vi "Config Ackermann Frame.vi"(10 "subpanel to main command event":T1, 11 "main to subpanel command event reg":T2) -> ()   [LabVIEW 2017, in "NI_Robotics_Configure Steering Frame.lvlib" / "Ackermann Frame Subpanel.lvlib"]
uses:
  <vilib>/robotics/Dialog/Configure Steering Frame/Ackermann Frame Subpanel/Ackermann Frame Subpanel.lvlib
  <vilib>/robotics/Dialog/Configure Steering Frame/Main to Subpanel Command Event Reg.ctl
  <vilib>/robotics/Dialog/Configure Steering Frame/Main to Subpanel Command.ctl
  <vilib>/robotics/Steering/Steering Frame/NI_Robotics_Steering Frame.lvclass
  <vilib>/robotics/Dialog/Configure Steering Frame/Subpanel to Main Command Event.ctl
  <vilib>/robotics/Dialog/Configure Steering Frame/Subpanel to Main Command.ctl
  <vilib>/robotics/Dialog/Configure Steering Frame/Ackermann Frame Subpanel/FP Refs.ctl
  <vilib>/robotics/Steering/Ackermann Steering Frame/NI_Robotics_Ackermann Steering Frame.lvclass
  c:/Program Files (x86)/National Instruments/LabVIEW 2017/vi.lib/robotics/Steering/Steering Frame/NI_Robotics_Steering Frame.lvclass
  <vilib>/robotics/Steering/Steering Frame/NI_Robotics_Steering Frame.lvclass/NI_Robotics_Steering Frame.ctl
  <vilib>/robotics/Steering/Wheel/NI_Robotics_Wheel.lvclass/NI_Robotics_Wheel.ctl
  <vilib>/robotics/Steering/Ackermann Steering Frame/NI_Robotics_Ackermann Steering Frame.lvclass/NI_Robotics_Ackermann Steering Frame.ctl
  <vilib>/robotics/Dialog/Configure Steering Frame/Send Update Picture Command.vi
  <vilib>/robotics/Steering/Ackermann Steering Frame/Set Wheel Separations.vi
  <vilib>/robotics/Dialog/Configure Steering Frame/Generate Subpanel to Main Event.vi
  <vilib>/Utility/error.llb/Clear Errors.vi
  <vilib>/robotics/Steering/Ackermann Steering Frame/Wheel Separation to Frame Positions.vi
  <vilib>/robotics/Steering/Steering Frame/Reposition Wheels.vi
  <vilib>/robotics/Steering/Wheel/Update Steering to Wheel Frame Transform.vi
  <vilib>/Analysis/coordinate.llb/Wrap Angle.vi
  <vilib>/Analysis/coordinate.llb/Wrap Angle (scalar).vi
  <vilib>/robotics/Steering/Steering Frame/Set All Gear Ratio.vi
  <vilib>/robotics/Steering/Steering Frame/Set All Wheel Radius.vi
  <vilib>/robotics/Dialog/Configure Steering Frame/NI_Robotics_Configure Steering Frame.lvlib
panel:
  in  "Wheel Separation Length":dbl
  in  "Wheel Separation Width":dbl
  in  "Gear Ratio":dbl
  in  "Wheel Radius":dbl
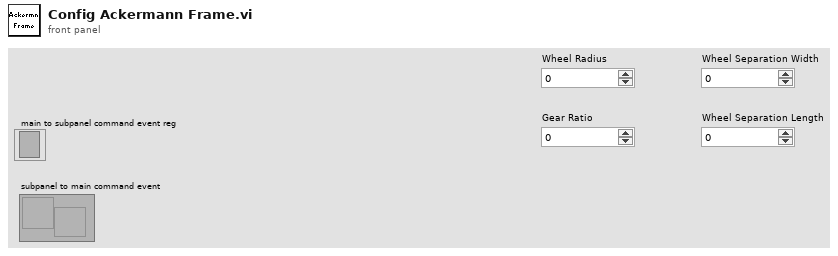
[diagram p1: front panel]
types:
  T1 = typedef "NI_Robotics_Configure Steering Frame.lvlib/Subpanel to Main Command Event.ctl" = refnum<user-event>
  T2 = typedef "NI_Robotics_Configure Steering Frame.lvlib/Main to Subpanel Command Event Reg.ctl" = refnum<event-registration>
  T3 = typedef "NI_Robotics_Configure Steering Frame.lvlib/Ackermann Frame Subpanel.lvlib/FP Refs.ctl" = cluster{"VI Refnum":refnum<vi>, "Wheel Radius":refnum<vi>, "Gear Ratio":refnum<vi>, "Wheel Separation Width":refnum<vi>, "Wheel Separation Length":refnum<vi>}
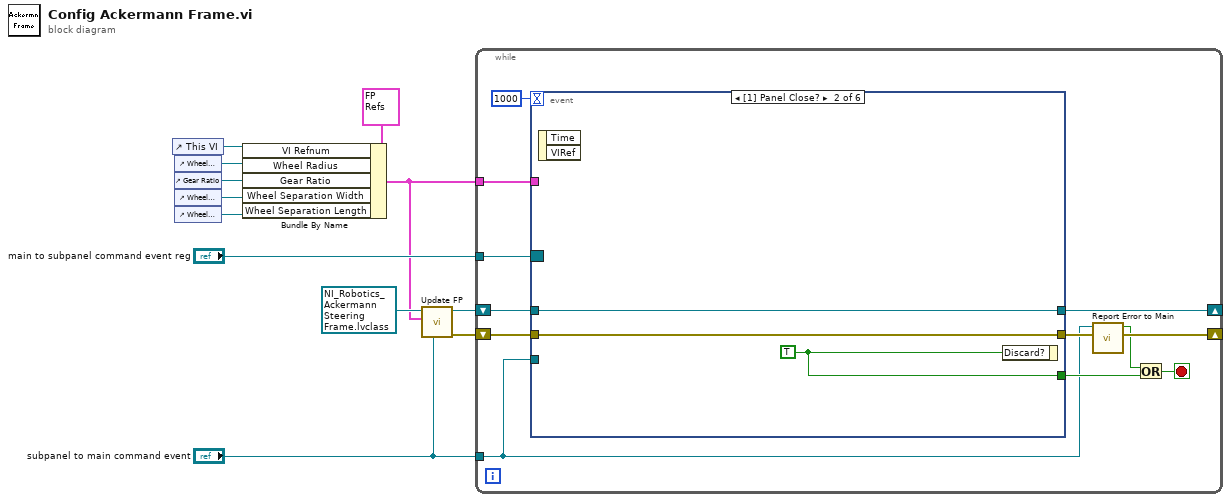
[diagram p0: block diagram]
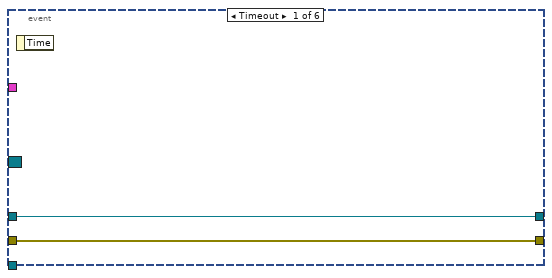
[diagram p2: hidden frame]
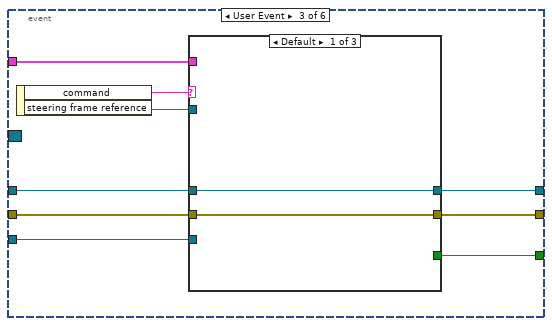
[diagram p3: hidden frame]
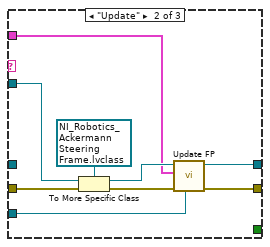
[diagram p4: hidden frame]
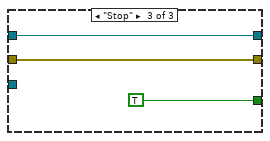
[diagram p5: hidden frame]
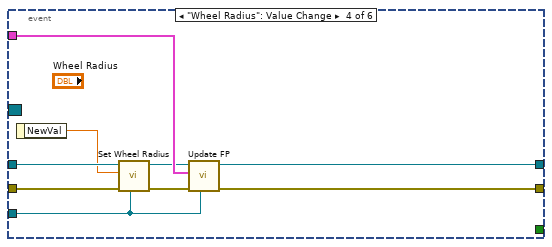
[diagram p6: hidden frame]
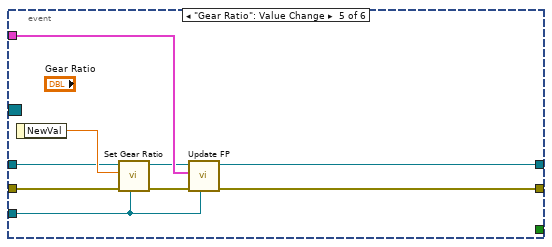
[diagram p7: hidden frame]
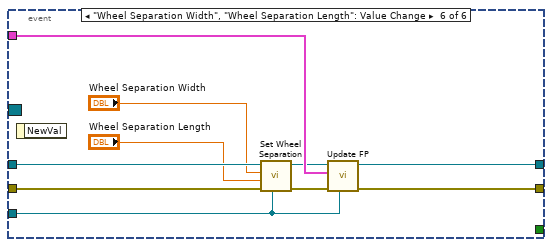
[diagram p8: hidden frame]
diagram:
  n1 = control-ref of="This VI"() -> (w11:refnum<vi>)
  n2 = control-ref of="Wheel Radius"() -> (w10:refnum<vi>)
  n3 = control-ref of="Gear Ratio"() -> (w9:refnum<vi>)
  n4 = control-ref of="Wheel Separation Width"() -> (w8:refnum<vi>)
  n5 = control-ref of="Wheel Separation Length"() -> (w7:refnum<vi>)
  n6 = Bundle By Name(cluster=T3 {"VI Refnum"=refnum, "Wheel Radius"=refnum, "Gear Ratio"=refnum, "Wheel Separation Width"=refnum, "Wheel Separation Length"=refnum} ("fp refs"), "VI Refnum"=w11, "Wheel Radius"=w10, "Gear Ratio"=w9, "Wheel Separation Width"=w8, "Wheel Separation Length"=w7) -> (w2:T3)
  n7 = call <vilib>:"Update FP.vi"("subpanel to main command event"="subpanel to main command event", "fp refs"=w2, "steering frame ref in"=refnum<data-value> refnum) -> ("error out"=w1:errorcluster, "steering frame ref out"=w4:refnum<data-value>)  [unwired: 7 in]
  n8 = while {
    tunnel: w2 -> [w23]
    tunnel: "main to subpanel command event reg" -> [w22]
    shift-right: [w20] -> _
    shift-left: w4 -> [w21]
    shift-right: [w18] -> _
    shift-left: w1 -> [w14]
    tunnel: "subpanel to main command event" -> [w13]
    stop <- w15 stop-if-true
    n9 = event shown="[1] Panel Close?" {
      selector: w22 -> [_ _ _ _ _ _]
      dyn-events: _ -> [_ _ _ _ _ _]
      timeout: 1000 -> [_ _ _ _ _ _]
      tunnel: w23 -> [_ _ w36 w59 w68 w78]
      tunnel: w21 -> [w26 w29 w35 w58 w66 w77]
      tunnel: [w26 w29 w34 w61 w70 w80] -> w20
      tunnel: [w25 w28 w33 w60 w69 w79] -> w19
      tunnel: [_ w27 w32 _ _ _] -> w17
      tunnel: w14 -> [w25 w28 w31 w55 w64 w75]
      tunnel: w13 -> [_ _ w30 w53 w62 w73]
      event Timeout {
        n10 = event-data() -> ()  [unwired: 1 in, 1 out]
      }
      event Panel Close? {
        w27 = TRUE ("Discard?")
        n11 = event-data() -> ()  [unwired: 1 in, 2 out]
        n12 = event-data("Discard?"=w27) -> ()  [unwired: 1 in, 1 out]
      }
      event User Event {
        n13 = event-data() -> ("command"=w38:string, "steering frame reference"=w37:refnum<data-value>)  [unwired: 1 in]
        n14 = case shown="Default" w38 {
          tunnel: w37 -> [_ w48 _]
          tunnel: w31 -> [w40 w47 w51]
          tunnel: [w40 w43 w51] -> w33
          tunnel: [w39 w45 w52] -> w34
          tunnel: w35 -> [w39 _ w52]
          tunnel: [_ _ TRUE] -> w32
          tunnel: w30 -> [_ w41 _]
          tunnel: w36 -> [_ w42 _]
          frame Default {
          }
          frame "Update" {
            n15 = To More Specific Class(target class=refnum<data-value> refnum ("data value reference"), reference=w48, error in=w47) -> (specific class reference=w46:refnum<data-value>, error out=w44:errorcluster)
            n16 = call <vilib>:"Update FP.vi"("subpanel to main command event"=w41, "error in (no error)"=w44, "fp refs"=w42, "steering frame ref in"=w46) -> ("error out"=w43:errorcluster, "steering frame ref out"=w45:refnum<data-value>)  [unwired: 6 in]
          }
          frame "Stop" {
          }
        }
      }
      event "Wheel Radius": Value Change {
        n17 = event-data() -> ("NewVal"=w56:dbl)  [unwired: 1 in]
        n18 = call <vilib>:"Set Wheel Radius.vi"("subpanel to main command event"=w53, "error in (no error)"=w55, "wheel radius"=w56, "steering frame ref in"=w58) -> ("error out"=w54:errorcluster, "steering frame ref out"=w57:refnum<data-value>)  [unwired: 6 in]
        n19 = call <vilib>:"Update FP.vi"("subpanel to main command event"=w53, "error in (no error)"=w54, "fp refs"=w59, "steering frame ref in"=w57) -> ("error out"=w60:errorcluster, "steering frame ref out"=w61:refnum<data-value>)  [unwired: 6 in]
      }
      event "Gear Ratio": Value Change {
        n20 = event-data() -> ("NewVal"=w67:dbl)  [unwired: 1 in]
        n21 = call <vilib>:"Set Gear Ratio.vi"("subpanel to main command event"=w62, "error in (no error)"=w64, "gear ratio"=w67, "steering frame ref in"=w66) -> ("error out"=w63:errorcluster, "steering frame ref out"=w65:refnum<data-value>)  [unwired: 6 in]
        n22 = call <vilib>:"Update FP.vi"("subpanel to main command event"=w62, "error in (no error)"=w63, "fp refs"=w68, "steering frame ref in"=w65) -> ("error out"=w69:errorcluster, "steering frame ref out"=w70:refnum<data-value>)  [unwired: 6 in]
      }
      event "Wheel Separation Width", "Wheel Separation Length": Value Change {
        n23 = event-data() -> ()  [unwired: 1 in, 1 out]
        n24 = call <vilib>:"Set Wheel Separation.vi"("subpanel to main command event"=w73, "error in (no error)"=w75, "wheel separation length"="Wheel Separation Length", "wheel separation width"="Wheel Separation Width", "steering frame ref in"=w77) -> ("error out"=w74:errorcluster, "steering frame ref out"=w76:refnum<data-value>)  [unwired: 5 in]
        n25 = call <vilib>:"Update FP.vi"("subpanel to main command event"=w73, "error in (no error)"=w74, "fp refs"=w78, "steering frame ref in"=w76) -> ("error out"=w79:errorcluster, "steering frame ref out"=w80:refnum<data-value>)  [unwired: 6 in]
      }
    }
    n26 = call <vilib>:"Report Error to Main.vi"("error in (no error)"=w19, "subpanel to main command event"=w13) -> ("error out"=w18:errorcluster, "reported error?"=w16:bool)  [unwired: 8 in]
    n27 = Or(x=w16, y=w17) -> (x .or. y?=w15:bool)
  }
